vi "Bloch Sphere - Read.vi"(7 "QuWire in":refnum<class "QuWire.lvclass">) -> (3 "x":dbl, 4 "y":dbl, 6 "z":dbl, 8 "r":dbl, 10 "theta":dbl, 15 "phi":dbl)   [LabVIEW 2020]
uses:
  QuSim/QuWire/QuWire.lvclass
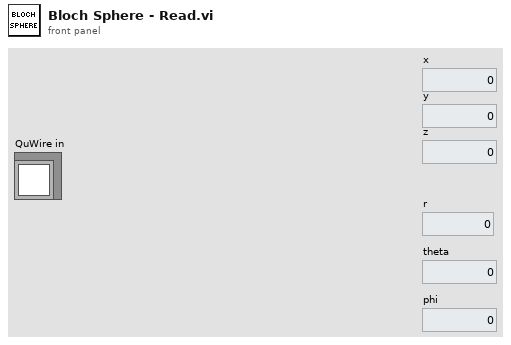
[diagram p1: front panel]
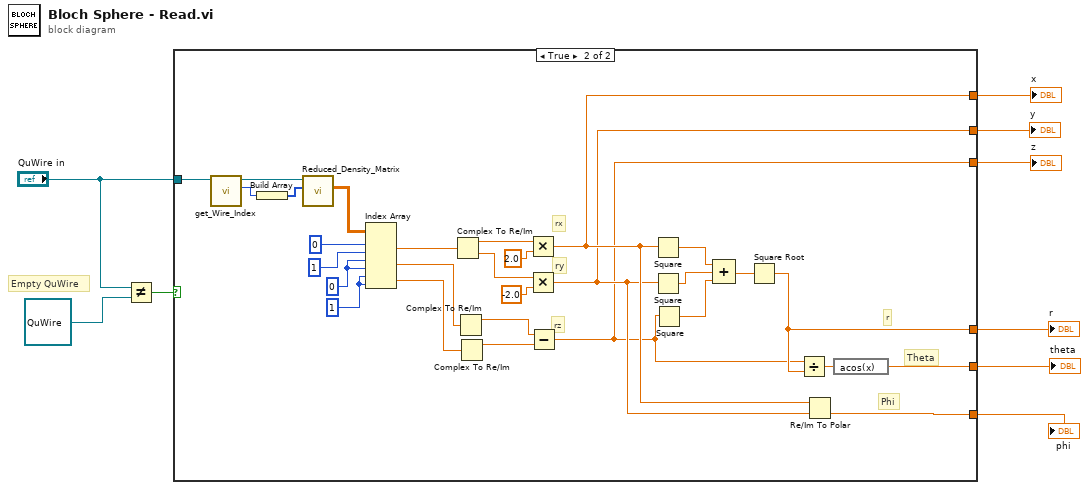
[diagram p0: block diagram]
diagram:
  # "Empty QuWire"
  n1 = Not Equal?(x="QuWire in", y=refnum<class "QuWire.lvclass"> refnum ("QuWire in")) -> (x != y?=w7:bool)
  n2 = case shown="True" w7 {
    tunnel: "QuWire in" -> [_ w19]
    tunnel: [_ w18] -> w6
    tunnel: [_ w17] -> w5
    tunnel: [_ w16] -> w4
    tunnel: [_ w15] -> w3
    tunnel: [_ w14] -> w2
    tunnel: [_ w13] -> w1
    frame False {
    }
    frame True {
      w35 = 1 ("disabled index (col)")
      w36 = 0 ("index (row)")
      # "Phi"
      # "Theta"
      # "r"
      # "rz"
      # "ry"
      # "rx"
      n3 = call "get_Wire_Index.vi"("QuWire in"=w19) -> ("Wire Index"=w11:i32, "QuWire out"=w12:refnum<class "QuWire.lvclass">)  [unwired: 8 in, 1 out]
      n4 = Build Array(w11) -> (w10:i32[])
      n5 = call "Reduced_Density_Matrix.vi"("Qubits to Keep"=w10, "QuWire in"=w12) -> ("Reduced Density Matrix"=w20:cdb[][])  [unwired: 6 in, 3 out]
      n6 = Index Array(array=w20, index (row) #1=0 ("index (row)"), index (col) #1=1 ("disabled index (col)"), index (row) #2=w36, index (col) #2=w36, index (row) #3=w35, index (col) #3=w35) -> (element #1=w34:cdb, element #2=w28:cdb, element #3=w27:cdb)
      n7 = Complex To Re/Im(x + iy=w34) -> (x=w33:dbl, y=w30:dbl)
      n8 = Complex To Re/Im(x + iy=w28) -> (x=w25:dbl)  [unwired: 1 out]
      n9 = Complex To Re/Im(x + iy=w27) -> (x=w26:dbl)  [unwired: 1 out]
      n10 = Multiply(x=w33, y=2.0) -> (x*y=w15:dbl)
      n11 = Multiply(x=w30, y=-2.0) -> (x*y=w14:dbl)
      n12 = Subtract(x=w25, y=w26) -> (x-y=w13:dbl)
      n13 = Square(x=w15) -> (x^2=w22:dbl)
      n14 = Square(x=w14) -> (x^2=w21:dbl)
      n15 = Square(x=w13) -> (x^2=w29:dbl)
      n16 = Compound Arithmetic op=ADD(w22, w21, w29) -> (w24:dbl)
      n17 = Square Root(x=w24) -> (sqrt(x)=w18:dbl)
      n18 = Divide(x=w13, y=w18) -> (x/y=w23:dbl)
      n19 = Re/Im To Polar(2:w14, 3:w15) -> (0:w16:dbl)  [unwired: 1 out]
      n20 = expression code="acos(x)"(w23) -> (w17:dbl)
    }
  }
  "r" <- w6
  "theta" <- w5
  "phi" <- w4
  "x" <- w3
  "y" <- w2
  "z" <- w1
